vi "Close.vi"(0 "VISA Resource Name":refnum<visa-resource-name>, 11 "error in (no error)":errorcluster {"code" format="%.0x"}) -> (15 "error out":errorcluster {"code" format="%.0x"})   [LabVIEW 2020, in "Olympus IX BX Series.lvlib"]
doc: "Closes the I/O interface."
uses:
  Olympus IX BX Series.lvlib
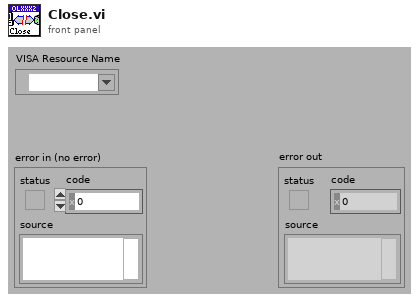
[diagram p1: front panel]
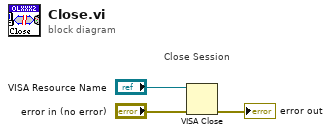
[diagram p0: block diagram]
diagram:
  # "Close Session"
  n1 = VISA Close(VISA resource name="VISA Resource Name", error in (no error)="error in (no error)") -> (error out=→"error out":errorcluster)
